vi "Configure test.vi"(6 "Assert VI Path":path, 7 "Existing Queue Elements":string, 8 "error in (no error)":errorcluster, 11 "Basic String in":refnum<class "String.lvclass">) -> (0 "error out":errorcluster, 3 "Basic String out":refnum<class "String.lvclass">)   [LabVIEW 2018, in "String.lvclass"]
uses:
  String.lvclass
  a9d232d7-dc99-4600-9e24-392b3dc17f67.vi
  <vilib>/JDP Science/JSONtext/Find Item.vi
  a9d232d7-dc99-4600-9e24-392b3dc17f67.vi/6dec4510-f9fd-4dda-805c-a9908ad8231b.vi
  a9d232d7-dc99-4600-9e24-392b3dc17f67.vi/e536fe6e-531a-41d7-9bfb-2a64022aad0e.vi
  <vilib>/JDP Science/JSONtext/String Subset.vi
  Test Class String IDs.vi
  <vilib>/JDP Science/JSONtext/Parsing/Parse Full Path or Item Name.vi
  <vilib>/JDP Science/JSONtext/Offset/Find Item Locations by Path.vi
  <vilib>/JDP Science/JSONtext/JSON text to Variant.vi
  <vilib>/JDP Science/JSONtext/Variant to JSON Text.vi
  <vilib>/JDP Science/JSONtext/Set Item.vi
  Test.lvclass
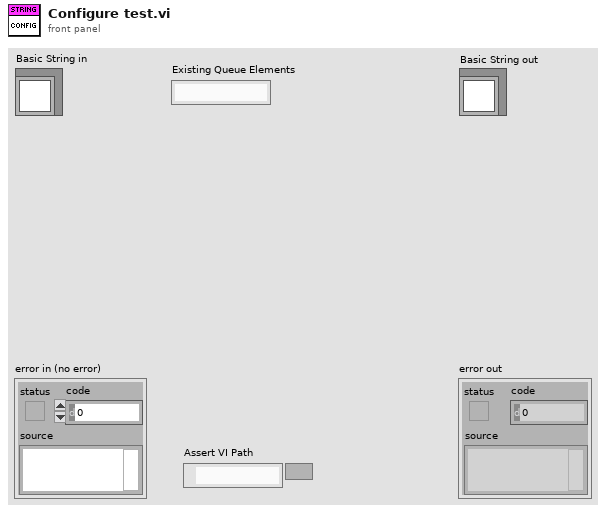
[diagram p1: front panel]
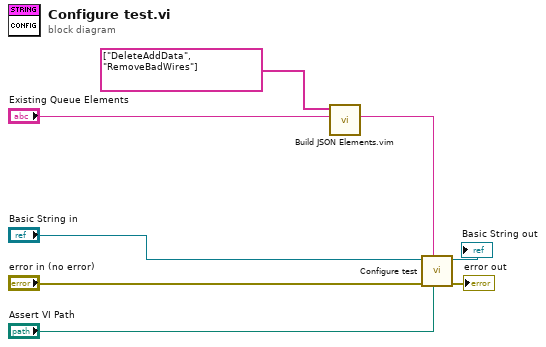
[diagram p0: block diagram]
diagram:
  n1 = call "Build JSON Elements.vim"("JSON Elements in ({})"="Existing Queue Elements", "Prepend Element(s)"=string[] ["DeleteAddData", "RemoveBadWires"]) -> ("JSON Elements out"=w1:string)  [unwired: 9 in]
  n2 = call-parent "Configure test.vi"("Assert VI Path"="Assert VI Path", "Existing Queue Elements"=w1, "error in (no error)"="error in (no error)", "Basic Test in"="Basic String in") -> ("error out"=→"error out":errorcluster, "Test out"=→"Basic String out":refnum<class "String.lvclass">)  [unwired: 6 in]
